vi "PSVCH_Custom Error.vi"(8 "error in (no error)":errorcluster, 10 "Source":string, 11 "Custom Code":i32) -> (0 "error out":errorcluster, 2 "Explanation":string, 3 "Custom Code":i32)   [LabVIEW 2016]
panel:
  in  "Error Code":i32
  in  "Source In":string
  out "Source Out":string
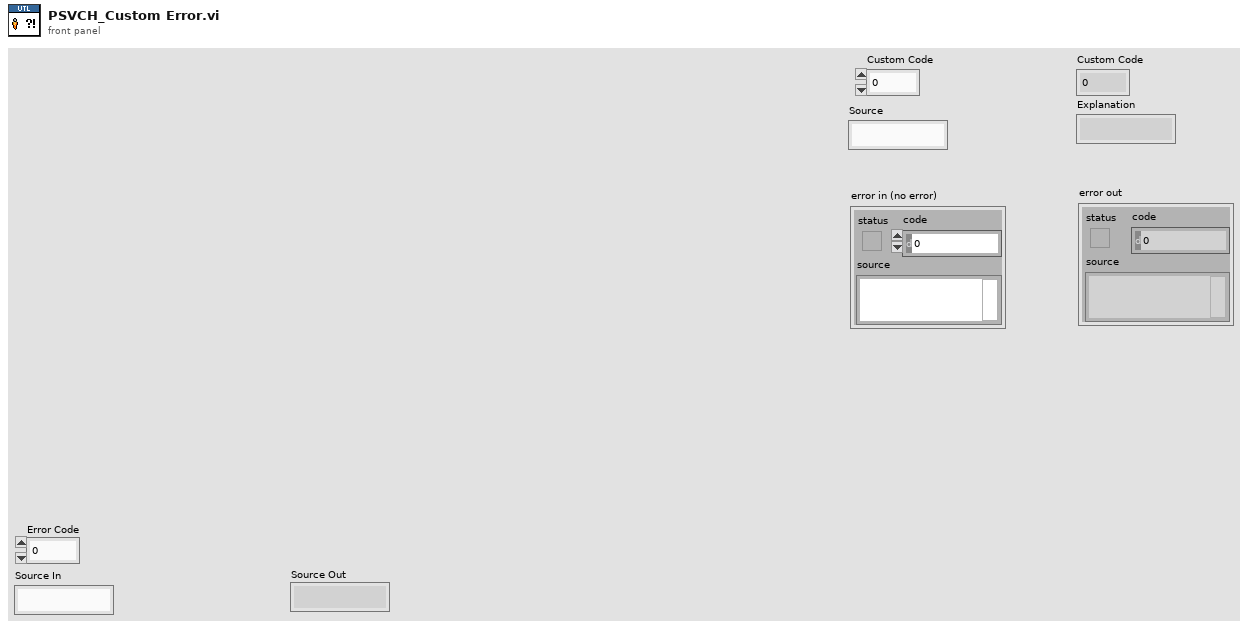
[diagram p1: front panel]
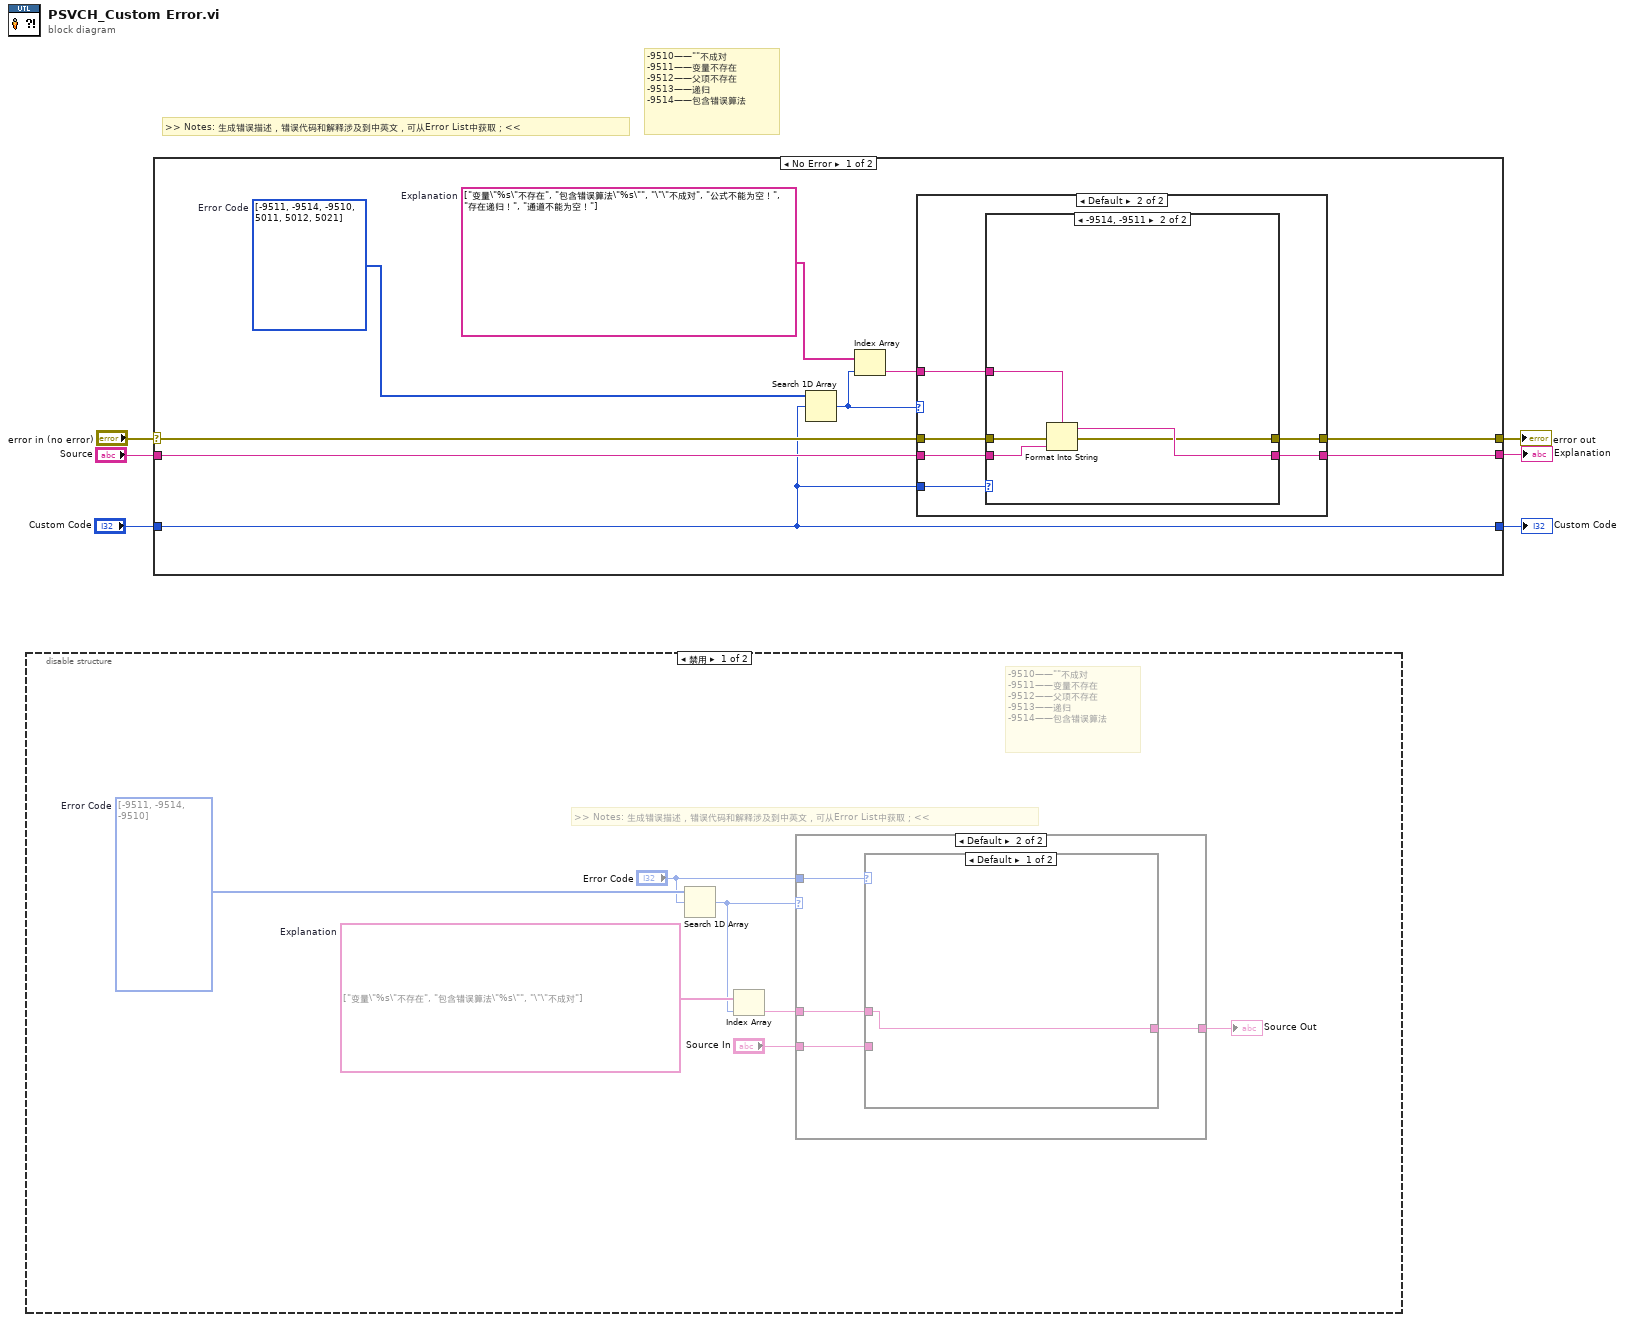
[diagram p0: block diagram]
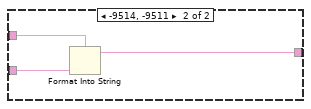
[diagram p3: hidden frame]
diagram:
  # "-9510——\"\"不成对\n-9511——变量不存在\n-9512——父项不存在\n-9513——递归\n-9514——包含错误算法"
  # ">> Notes: 生成错误描述，错误代码和解释涉及到中英文，可从Error List中获取；<<"
  n1 = disable-structure shown="禁用" {
    frame Disabled {
      w13 = string[] ["变量\"%s\"不存在", "包含错误算法\"%s\"", "\"\"不成对"]  # Explanation
      w8 = i32[] [-9511, -9514, -9510]  # Error Code
      # "-9510——\"\"不成对\n-9511——变量不存在\n-9512——父项不存在\n-9513——递归\n-9514——包含错误算法"
      # ">> Notes: 生成错误描述，错误代码和解释涉及到中英文，可从Error List中获取；<<"
      n2 = Search 1D Array(1D array=w8, element="Error Code") -> (index of element=w9:i32)  [unwired: 1 in]
      n3 = Index Array(array=w13, index=w9) -> (element=w12:string)
      n4 = case shown="Default" w9 {
        tunnel: "Error Code" -> [_ w18]
        tunnel: w12 -> [_ w17]
        tunnel: "Source In" -> [w14 w16]
        tunnel: [w14 w15] -> w10
        frame -1 {
        }
        frame Default {
          n5 = case shown="Default" w18 {
            tunnel: w17 -> [w19 w22]
            tunnel: w16 -> [_ w21]
            tunnel: [w19 w20] -> w15
            frame Default {
            }
            frame -9514, -9511 {
              n6 = Format Into String(format string=w22, w21) -> (resulting string=w20:string)  [unwired: 2 in, 1 out]
            }
          }
        }
      }
      "Source Out" <- w10
    }
    frame Enabled {
    }
  }
  n7 = case shown="No Error" "error in (no error)" {
    selector: "error in (no error)" -> [w27 w47]
    tunnel: [w25 w47] -> w6
    tunnel: "Custom Code" -> [w24 _]
    tunnel: "Source" -> [w28 _]
    tunnel: [w24 _] -> w2
    tunnel: [w23 _] -> w1
    frame No Error {
      w29 = string[] ["变量\"%s\"不存在", "包含错误算法\"%s\"", "\"\"不成对", "公式不能为空！", "存在递归！", "通道不能为空！"]  # Explanation
      w26 = i32[] [-9511, -9514, -9510, 5011, 5012, 5021]  # Error Code
      n8 = Search 1D Array(1D array=w26, element=w24) -> (index of element=w31:i32)  [unwired: 1 in]
      n9 = Index Array(array=w29, index=w31) -> (element=w30:string)
      n10 = case shown="Default" w31 {
        tunnel: w24 -> [_ w39]
        tunnel: w30 -> [_ w38]
        tunnel: w28 -> [w33 w37]
        tunnel: [w33 w36] -> w23
        tunnel: w27 -> [w32 w35]
        tunnel: [w32 w34] -> w25
        frame -1 {
        }
        frame Default {
          n11 = case shown="-9514, -9511" w39 {
            tunnel: w38 -> [w41 w46]
            tunnel: w37 -> [_ w45]
            tunnel: [w41 w44] -> w36
            tunnel: w35 -> [w40 w43]
            tunnel: [w40 w42] -> w34
            frame Default {
            }
            frame -9514, -9511 {
              n12 = Format Into String(format string=w46, error in=w43, w45) -> (resulting string=w44:string, error out=w42:errorcluster)  [unwired: 1 in]
            }
          }
        }
      }
    }
    frame Error {
    }
  }
  "error out" <- w6
  "Custom Code" <- w2
  "Explanation" <- w1
